vi "StopPowerMonitor.vi"(8 "error in (no error)":errorcluster, 11 "handle":u64) -> (0 "error out":errorcluster)   [LabVIEW 2015, in "ReDeX.lvlib"]
doc: "redex_lv_result redex_lv_start_measurement(redex_lv_handle handle);"
uses:
  ReDeX.lvlib
  ReDeX.dll
panel:
  out "function return":u32(ring)
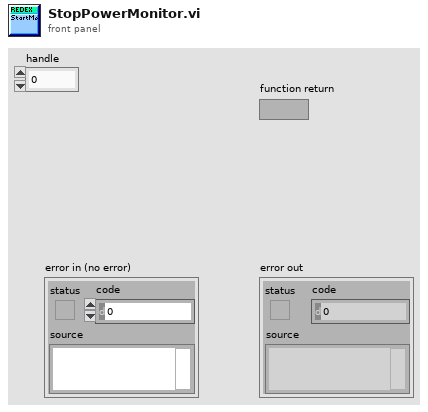
[diagram p1: front panel]
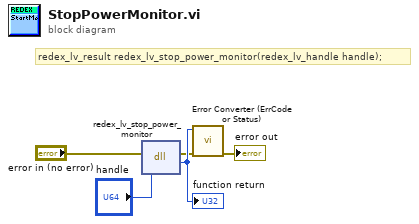
[diagram p0: block diagram]
diagram:
  # "redex_lv_result redex_lv_stop_power_monitor(redex_lv_handle handle);"
  n1 = dll-call lib="C:/Users/Marcel Hasler/Desktop/ReDeX 1.0pre3/LabVIEW/ReDeX.dll" fn="redex_lv_stop_power_monitor"(error in="error in (no error)", "handle"="handle") -> (error out=w3:errorcluster, "return type"=w5:u32)  [unwired: 3 in, 1 out]
  "function return" <- w5
  n2 = call "Error Converter (ErrCode or Status).vi"("error in (no error)"=w3, "error code"=w5) -> ("error out"=→"error out":errorcluster)  [unwired: 9 in]
